vi "instrument.PPMS1.TestLauncher.vi"() -> ()   [LabVIEW 2016, in "instrument.PPMS1.lvclass"]
uses:
  instrument.PPMS1.lvclass
  <vilib>/JKI/JKI SMO/SMO/Typedefs/SMOState --Enum.ctl
  C:/Program Files (x86)/National Instruments/LabVIEW 2016/vi.lib/JKI/JKI SMO/SMO/SMO.lvclass
  <vilib>/JKI/JKI SMO/SMO/SMO.lvclass
panel:
  in  "Debug Mode? [F]":bool
  out "SMO State":T1
  out "error out":errorcluster
  in  "Stop":bool
  # "PPMS1 Test Launcher"
  # "For instructions on how to use the JKI State Machine Objects, examples and video tutorials, visit:\nhttp://jki.net/state-machine-objects/\n\nJKI State Machine Objects™\nhttp://jki.net/state-machine-objects/\nCopyright (C) 2005-2015, JKI <info@jki.net>\nALL RIGHTS RESERVED"
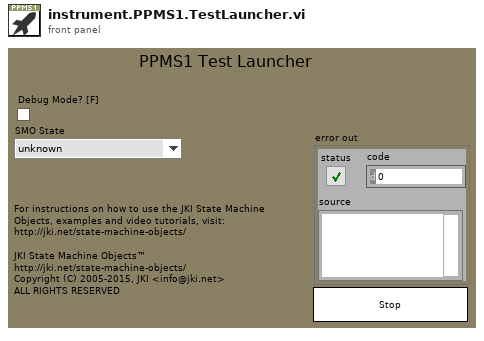
[diagram p1: front panel]
types:
  T1 = typedef "SMO.lvclass/SMOState --Enum.ctl" = enum16{"unknown", "Created", "Started", "Stopped"}
  T2 = typedef "SMO.lvclass/Public Events.ctl" = cluster{"Error":refnum<user-event>, "State":refnum<user-event>, "Reserve State":refnum<user-event>}
  T3 = cluster{"Event Registration Refnum":refnum<event-registration>}
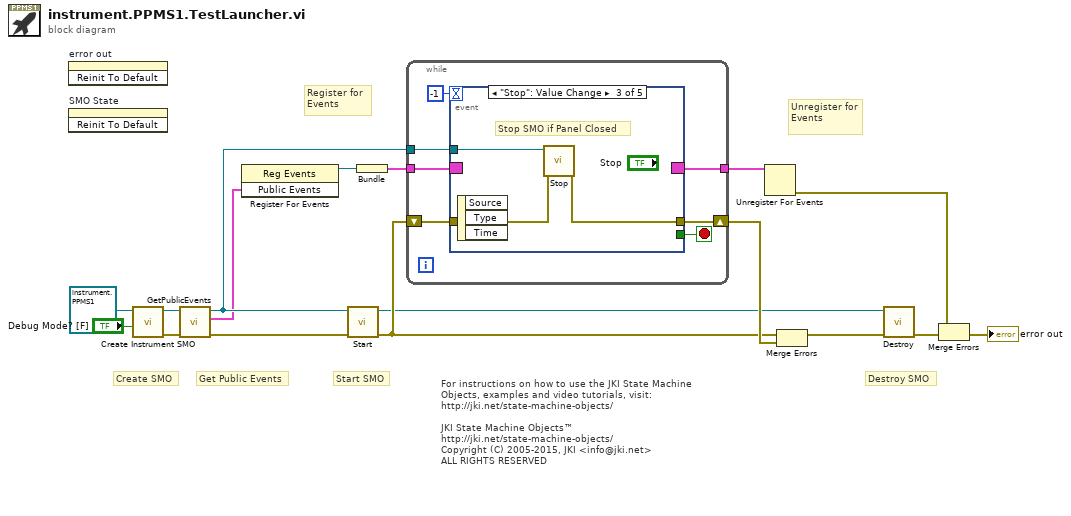
[diagram p0: block diagram]
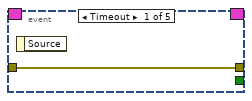
[diagram p2: hidden frame]
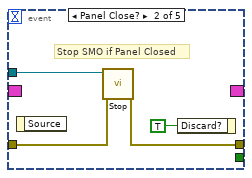
[diagram p3: hidden frame]
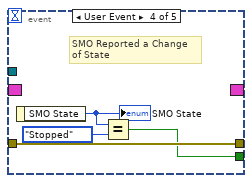
[diagram p4: hidden frame]
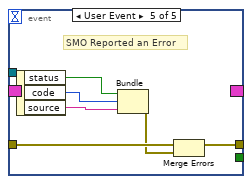
[diagram p5: hidden frame]
diagram:
  # "For instructions on how to use the JKI State Machine Objects, examples and video tutorials, visit:\nhttp://jki.net/state-machine-objects/\n\nJKI State Machine Objects™\nhttp://jki.net/state-machine-objects/\nCopyright (C) 2005-2015, JKI <info@jki.net>\nALL RIGHTS RESERVED"
  # "Get Public Events"
  # "Start SMO"
  # "Destroy SMO"
  # "Create SMO"
  # "Unregister for Events"
  # "Register for Events"
  n1 = invoke on="error out" class="Clust (strict)" method="Reinit To Default"() -> ()  [unwired: 3 in, 3 out]
  n2 = invoke on="SMO State" class="Enum (strict)" method="Reinit To Default"() -> ()  [unwired: 3 in, 3 out]
  n3 = call-dynamic "Create Instrument SMO.vi"("Debug Mode? [F]"="Debug Mode? [F]", "Instrument in"=refnum<class "instrument.PPMS1.lvclass"> refnum ("SMO.Template.lvclass")) -> ("error out"=w6:errorcluster, "Instrument out"=w7:refnum<class "instrument.PPMS1.lvclass">)  [unwired: 8 in]
  n4 = call <vilib>:"GetPublicEvents.vi"("error in (no error)"=w6, "SMO"=w7) -> ("error out"=w5:errorcluster, "Public Events"=w3:T2, "SMO out"=w4:refnum<class "instrument.PPMS1.lvclass">)  [unwired: 7 in]
  n5 = register-events(w3) -> (reference out=w2:refnum<event-registration>)  [unwired: 2 in, 1 out]
  n6 = call <vilib>:"Start.vi"("error in (no error)"=w5, "SMO"=w4) -> ("error out"=w10:errorcluster, "SMO out"=w8:refnum<class "instrument.PPMS1.lvclass">)  [unwired: 8 in]
  n7 = Bundle("Event Registration Refnum"=w2) -> (w16:T3)  [unwired: 1 in]
  n8 = while {
    shift-right: [w23] -> w15
    shift-left: w10 -> [w22]
    tunnel: w16 -> [w21]
    tunnel: [w20] -> w17
    tunnel: w4 -> [w19]
    stop <- w24 stop-if-true
    n9 = event shown="[2] \"Stop\": Value Change" {
      selector: w21 -> [_ _ _ _ _]
      dyn-events: [_ _ _ _ _] -> w20
      timeout: -1 -> [_ _ _ _ _]
      tunnel: [_ _ _ w33 _] -> w24
      tunnel: w19 -> [_ w29 w32 _ _]
      tunnel: [w25 w28 w31 w36 w40] -> w23
      tunnel: w22 -> [w25 w27 w30 w36 w38]
      event Timeout {
        n10 = event-data() -> ()  [unwired: 1 in, 1 out]
      }
      event Panel Close? {
        # "Stop SMO if Panel Closed"
        n11 = event-data() -> ()  [unwired: 1 in, 1 out]
        n12 = call <vilib>:"Stop.vi"("error in (no error)"=w27, "SMO"=w29) -> ("error out"=w28:errorcluster)  [unwired: 8 in, 1 out]
        n13 = event-data("Discard?"=TRUE ("OK")) -> ()  [unwired: 1 in, 1 out]
      }
      event "Stop": Value Change {
        # "Stop SMO if Panel Closed"
        n14 = event-data() -> ()  [unwired: 1 in, 3 out]
        n15 = call <vilib>:"Stop.vi"("error in (no error)"=w30, "SMO"=w32) -> ("error out"=w31:errorcluster)  [unwired: 8 in, 1 out]
      }
      event User Event {
        # "SMO Reported a Change\nof State"
        n16 = event-data() -> ("SMO State"=w35:T1)  [unwired: 1 in]
        "SMO State" <- w35
        n17 = Equal?(x=w35, y=SMOState_--Enum."Stopped") -> (x = y?=w33:bool)
      }
      event User Event {
        # "SMO Reported an Error"
        n18 = event-data() -> ("status"=w39:bool, "code"=w42:i32, "source"=w41:string)  [unwired: 1 in]
        n19 = Bundle("status"=w39, "code"=w42, "source"=w41) -> (w37:errorcluster)  [unwired: 1 in]
        n20 = Merge Errors(w38, w37) -> (w40:errorcluster)
      }
    }
  }
  n21 = Unregister For Events(event registration refnum=w17) -> (error out=w14:errorcluster)  [unwired: 1 in]
  n22 = Merge Errors(w10, w15) -> (w9:errorcluster)
  n23 = call <vilib>:"Destroy.vi"("error in (no error)"=w9, "SMO"=w8) -> ("error out"=w12:errorcluster)  [unwired: 9 in]
  n24 = Merge Errors(w14, w12) -> (→"error out":errorcluster)
